vi "EXO设置.vi"() -> ()   [LabVIEW 2016, in "main.lvlib"]
uses:
  main.lvlib
  control/checkbox.ctl
panel:
  in  "盐度":T1
  in  "蓝绿藻":T1
  in  "保存":bool
  in  "叶绿素a":T1
  in  "浊度":T1
  in  "DO":T1
  in  "ORP":T1
  in  "pH":T1
  in  "电导率":T1
  in  "水温":T1
  in  "EXO2是否存单表":T1
  in  "电导率系数":dbl=1.0
  in  "电导率单位":enum16{"μS/cm", "mS/cm"}(ring)
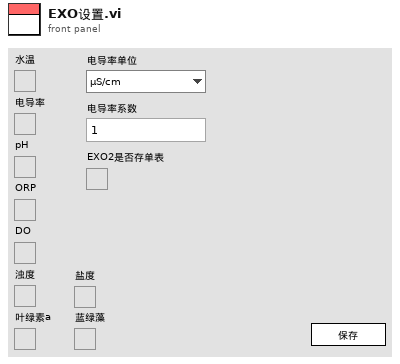
[diagram p1: front panel]
types:
  T1 = typedef "checkbox.ctl" = bool
  T2 = cluster{"水温":T1, "电导率":T1, "pH":T1, "ORP":T1, "DO":T1, "浊度":T1, "叶绿素a":T1, "蓝绿藻":T1, "盐度":T1}
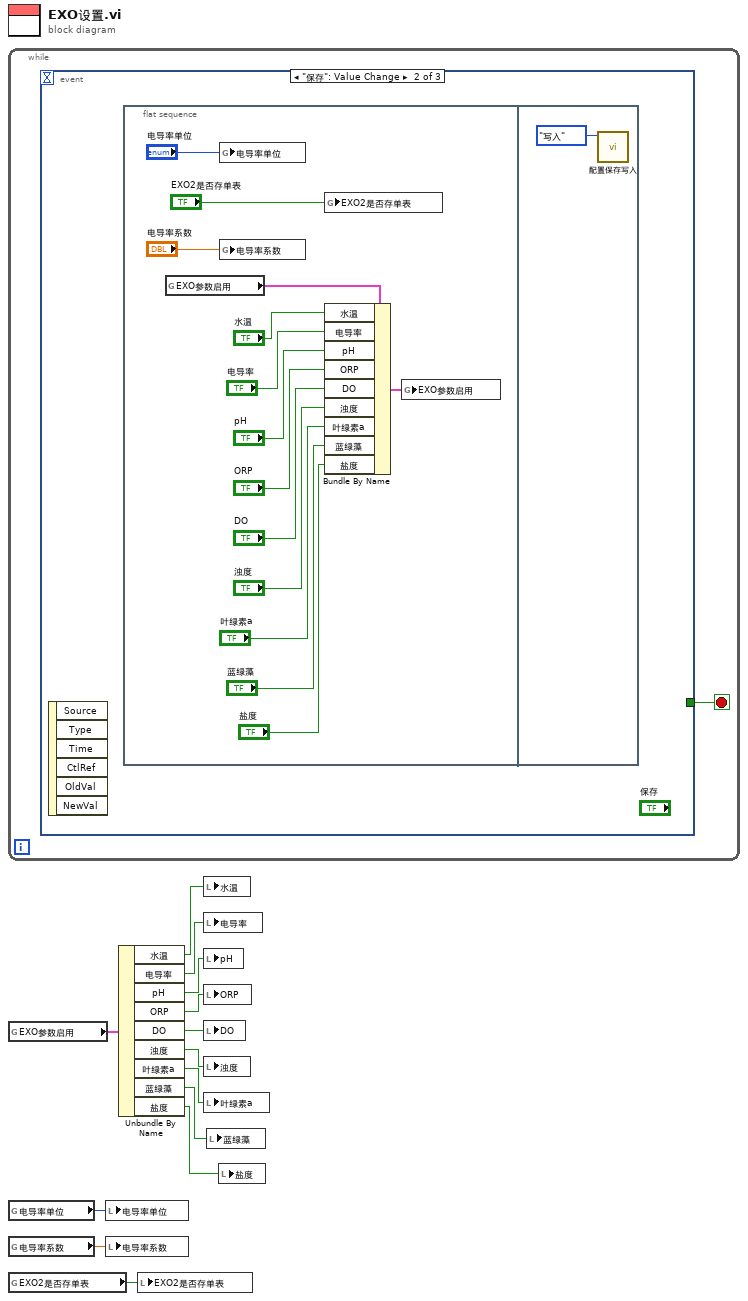
[diagram p0: block diagram]
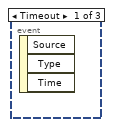
[diagram p2: hidden frame]
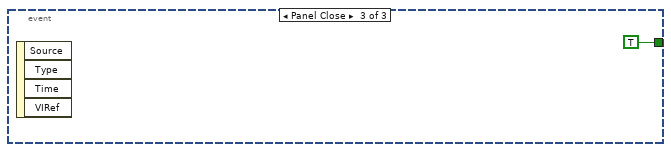
[diagram p3: hidden frame]
diagram:
  n1 = while {
    stop <- w14 stop-if-true
    n2 = event shown="[1] \"保存\": Value Change" {
      selector: _ -> [_ _ _]
      dyn-events: _ -> [_ _ _]
      timeout: _ -> [_ _ _]
      tunnel: [_ _ TRUE] -> w14
      event Timeout {
        n3 = event-data() -> ()  [unwired: 1 in, 3 out]
      }
      event "保存": Value Change {
        n4 = event-data() -> ()  [unwired: 1 in, 6 out]
        n5 = flat-sequence {
          frame #0 {
            n6 = global read "全局断电保存变量.vi" "EXO参数启用"() -> (w28:T2)
            n7 = global write "全局断电保存变量.vi" "电导率单位"("电导率单位") -> ()
            n8 = global write "全局断电保存变量.vi" "电导率系数"("电导率系数") -> ()
            n9 = global write "全局断电保存变量.vi" "EXO2是否存单表"("EXO2是否存单表") -> ()
            n10 = Bundle By Name(cluster=w28, "水温"="水温", "电导率"="电导率", "pH"="pH", "ORP"="ORP", "DO"="DO", "浊度"="浊度", "叶绿素a"="叶绿素a", "蓝绿藻"="蓝绿藻", "盐度"="盐度") -> (w27:T2)
            n11 = global write "全局断电保存变量.vi" "EXO参数启用"(w27) -> ()
          }
          frame #1 {
            n12 = call "配置保存写入.vi"("配置"=enum16{"读取", "写入"}."写入") -> ()  [unwired: 10 in, 1 out]
          }
        }
      }
      event Panel Close {
        n13 = event-data() -> ()  [unwired: 1 in, 4 out]
      }
    }
  }
  n14 = global read "全局断电保存变量.vi" "EXO参数启用"() -> (w13:T2)
  n15 = global read "全局断电保存变量.vi" "电导率单位"() -> (w4:enum16{"μS/cm", "mS/cm"})
  n16 = global read "全局断电保存变量.vi" "电导率系数"() -> (w5:dbl)
  n17 = global read "全局断电保存变量.vi" "EXO2是否存单表"() -> (w3:T1)
  n18 = local write "电导率单位"(w4) -> ()
  n19 = local write "电导率系数"(w5) -> ()
  n20 = Unbundle By Name(w13) -> ("水温"=w6:T1, "电导率"=w7:T1, "pH"=w8:T1, "ORP"=w9:T1, "DO"=w10:T1, "浊度"=w11:T1, "叶绿素a"=w12:T1, "蓝绿藻"=w2:T1, "盐度"=w1:T1)
  n21 = local write "EXO2是否存单表"(w3) -> ()
  n22 = local write "水温"(w6) -> ()
  n23 = local write "电导率"(w7) -> ()
  n24 = local write "pH"(w8) -> ()
  n25 = local write "ORP"(w9) -> ()
  n26 = local write "DO"(w10) -> ()
  n27 = local write "浊度"(w11) -> ()
  n28 = local write "叶绿素a"(w12) -> ()
  n29 = local write "蓝绿藻"(w2) -> ()
  n30 = local write "盐度"(w1) -> ()
